vi "set_ref_clus_thcd401.vi"(6 "variable_ref":T1, 8 "FM1":dbl, 9 "FC2":dbl, 10 "FC1":dbl, 11 "status":bool) -> ()   [LabVIEW 2019]
uses:
  cluster_ref_thcd401.ctl
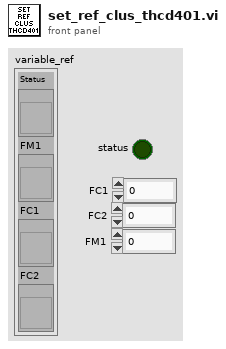
[diagram p1: front panel]
types:
  T1 = typedef "cluster_ref_thcd401.ctl" = cluster{"Status":refnum<vi>, "FM1":refnum<vi>, "FC1":refnum<vi>, "FC2":refnum<vi>}
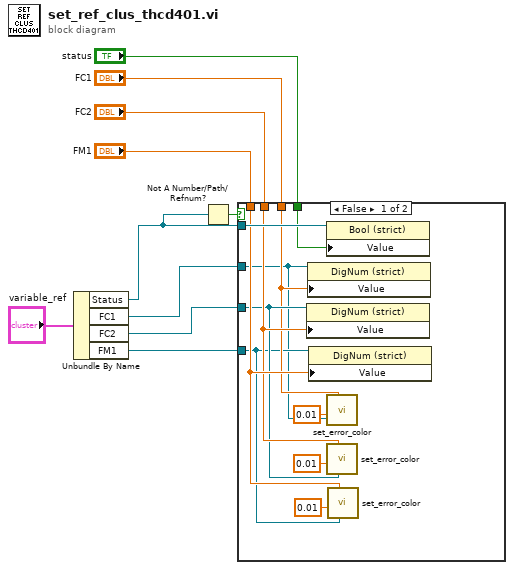
[diagram p0: block diagram]
diagram:
  n1 = Unbundle By Name("variable_ref") -> ("Status"=w6:refnum<vi>, "FC1"=w7:refnum<vi>, "FC2"=w8:refnum<vi>, "FM1"=w9:refnum<vi>)
  n2 = Not A Number/Path/Refnum?(number/path/refnum=w6) -> (NaN/Path/Refnum?=w10:bool)
  n3 = case shown="False" w10 {
    tunnel: "FC1" -> [w14 _]
    tunnel: "FC2" -> [w17 _]
    tunnel: "FM1" -> [w19 _]
    tunnel: w7 -> [w11 _]
    tunnel: w8 -> [w16 _]
    tunnel: w9 -> [w13 _]
    tunnel: w6 -> [w21 _]
    tunnel: "status" -> [w20 _]
    frame False {
      n4 = property class="DigNum (strict)"(reference=w16, "Value"=w17) -> ()  [unwired: 1 in, 2 out]
      n5 = property class="DigNum (strict)"(reference=w11, "Value"=w14) -> ()  [unwired: 1 in, 2 out]
      n6 = property class="DigNum (strict)"(reference=w13, "Value"=w19) -> ()  [unwired: 1 in, 2 out]
      n7 = property class="Bool (strict)"(reference=w21, "Value"=w20) -> ()  [unwired: 1 in, 2 out]
      n8 = call "set_error_color.vi"("value_ref"=w11, "value"=w14, "lo"=0.01) -> ()  [unwired: 9 in]
      n9 = call "set_error_color.vi"("value_ref"=w16, "value"=w17, "lo"=0.01) -> ()  [unwired: 9 in]
      n10 = call "set_error_color.vi"("value_ref"=w13, "value"=w19, "lo"=0.01) -> ()  [unwired: 9 in]
    }
    frame True {
    }
  }
